vi "Get SysDef Refnum (SubVI).vi"(8 "error in (no error)":errorcluster, 10 "System Definition path":path) -> (0 "error out":errorcluster, 3 "SysDef Refnum out":refnum<k24>)   [LabVIEW 2021, in "FPGA Addon Test Class.lvclass"]
uses:
  FPGA Addon Test Class.lvclass
  NationalInstruments.VeriStand.SystemDefinitionAPI
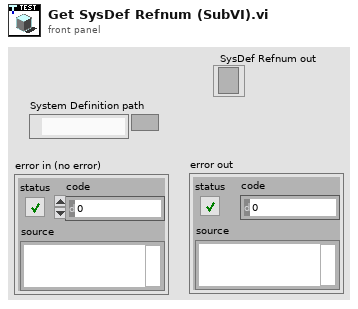
[diagram p1: front panel]
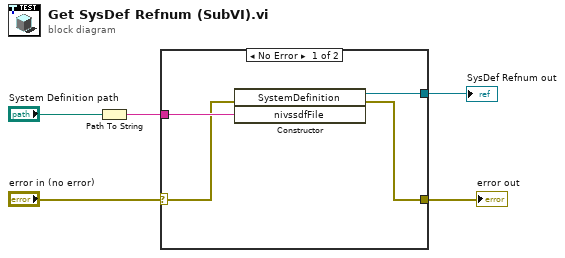
[diagram p0: block diagram]
diagram:
  n1 = Path To String(path="System Definition path") -> (string=w3:string)
  n2 = case shown="No Error" "error in (no error)" {
    selector: "error in (no error)" -> [w6 w10]
    tunnel: [w9 _] -> w5
    tunnel: [w8 w10] -> w4
    tunnel: w3 -> [w7 _]
    frame No Error {
      n3 = constructor class="SystemDefinition"(error in=w6, "nivssdfFile"=w7) -> (reference out=w9:refnum<k24>, error out=w8:errorcluster)  [unwired: 2 in, 2 out]
    }
    frame Error {
    }
  }
  "SysDef Refnum out" <- w5
  "error out" <- w4
